vi "QEPROcontrol_version3.vi"() -> ()   [LabVIEW 2014]
uses:
  C:/Program Files (x86)/Ocean Optics/OmniDriver/OOI_HOME/NETOmniDriver-NET40.dll
  <vilib>/ptbypt/NI_PtbyPt.lvlib
panel:
  out "CV值計算\n(100個取樣點)":dbl
  out "deltaR/R":dbl(graph)
  out "deltaR/R(%)":dbl
  out "max":dbl
  out "average":dbl
  out "x-y":dbl(graph)
  out "CVP波形(1/total R)\n全光譜加總取倒數":dbl(graph)
  in  "Record Number":i32 min=0 step=1
  in  "Record?":bool
  in  "Folder Path":path
  in  "Filename":string(combo)="RAtery"
  in  "stop":bool
  out "Spectrum":cluster{"Y":dbl[], "Y":dbl[]}[](graph)
  in  "Start/Pause":bool
  in  "TEC Enable":i16(ring)=1 items=["Disable", "Enable"]
  out "Detector\nTemperature":dbl
  in  "Enter the Detector\nTemperature (C)":dbl=-18.0
  in  "Scans to Average":i32=1 min=1 max=1000000 step=1
  out "Strobe Enable":i32(ring) items=["Disable", "Enable"]
  out "NumberOfPixels":i32
  out "NumberOfDarkPixels":i32
  in  "Correct for Electrical Dark":i16(ring) items=["Disable", "Enable"]
  in  "Correct for Detector Nonlinearity":i16(ring) items=["Disable", "Enable"]
  in  "BoxcarWidth":i32 min=0 max=1052 step=1
  out "Spectrometer ID":string
  in  "Integration\nTime (s.)":dbl=0.008 caption="Integration Time (s.)" min=0.008 max=60000.0 step=0.001 format="%#.6g"
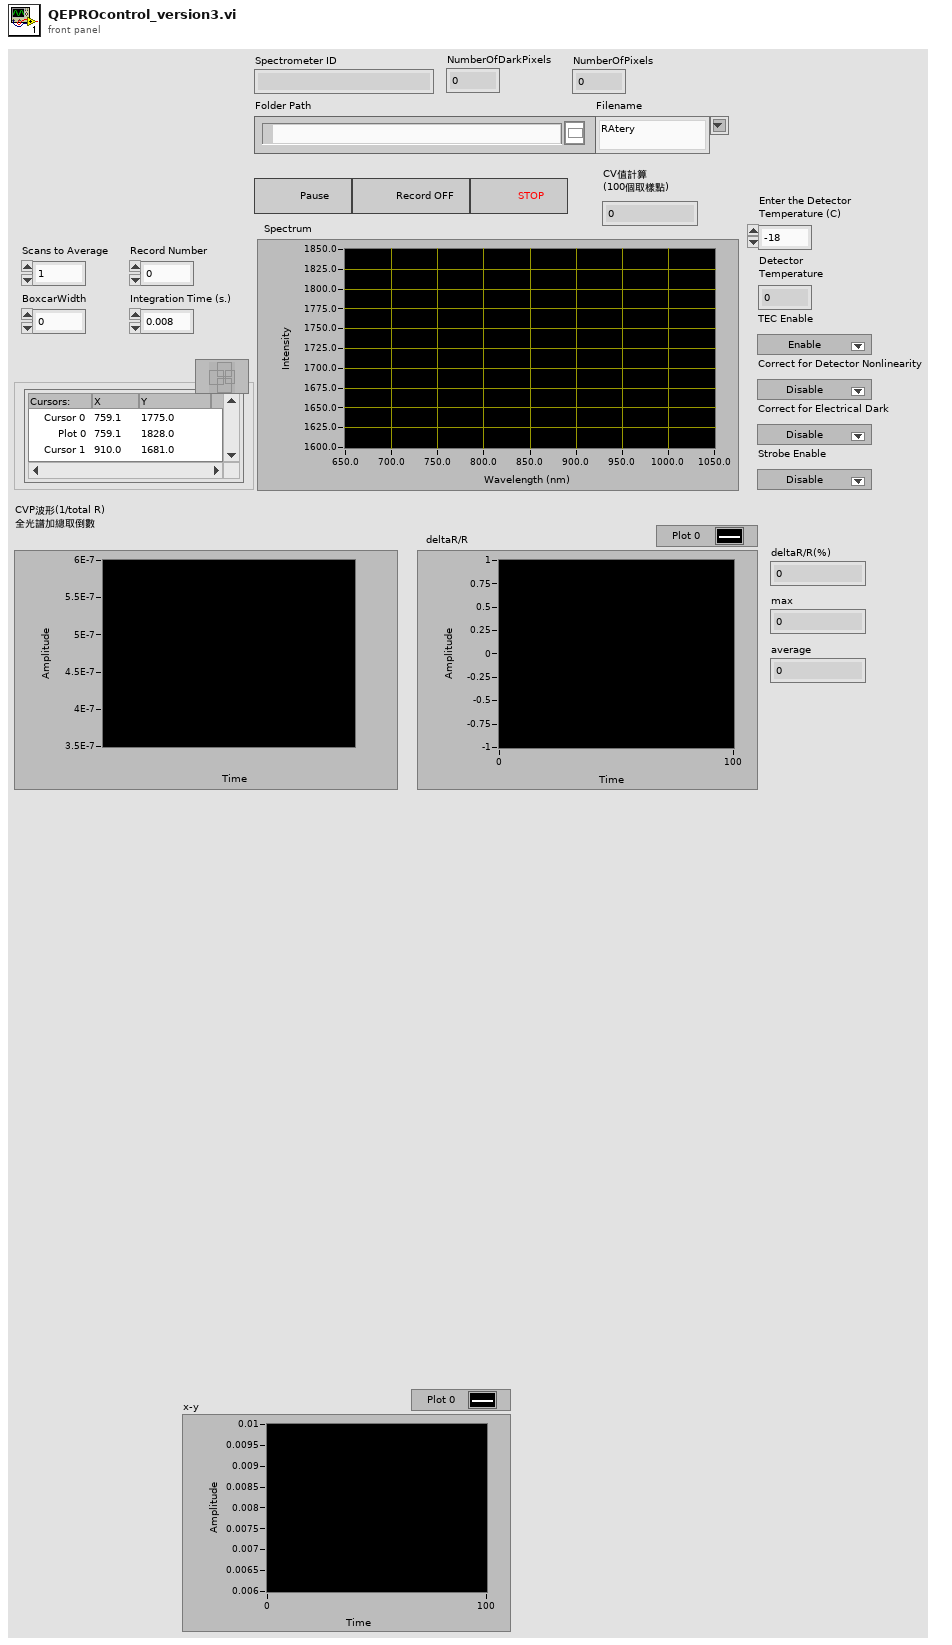
[diagram p1: front panel]
types:
  T1 = cluster{"seconds since 1Jan1904":timestamp, "getSpectrum":dbl[]}
  T2 = cluster{"seconds since 1Jan1904":timestamp, dbl[]}
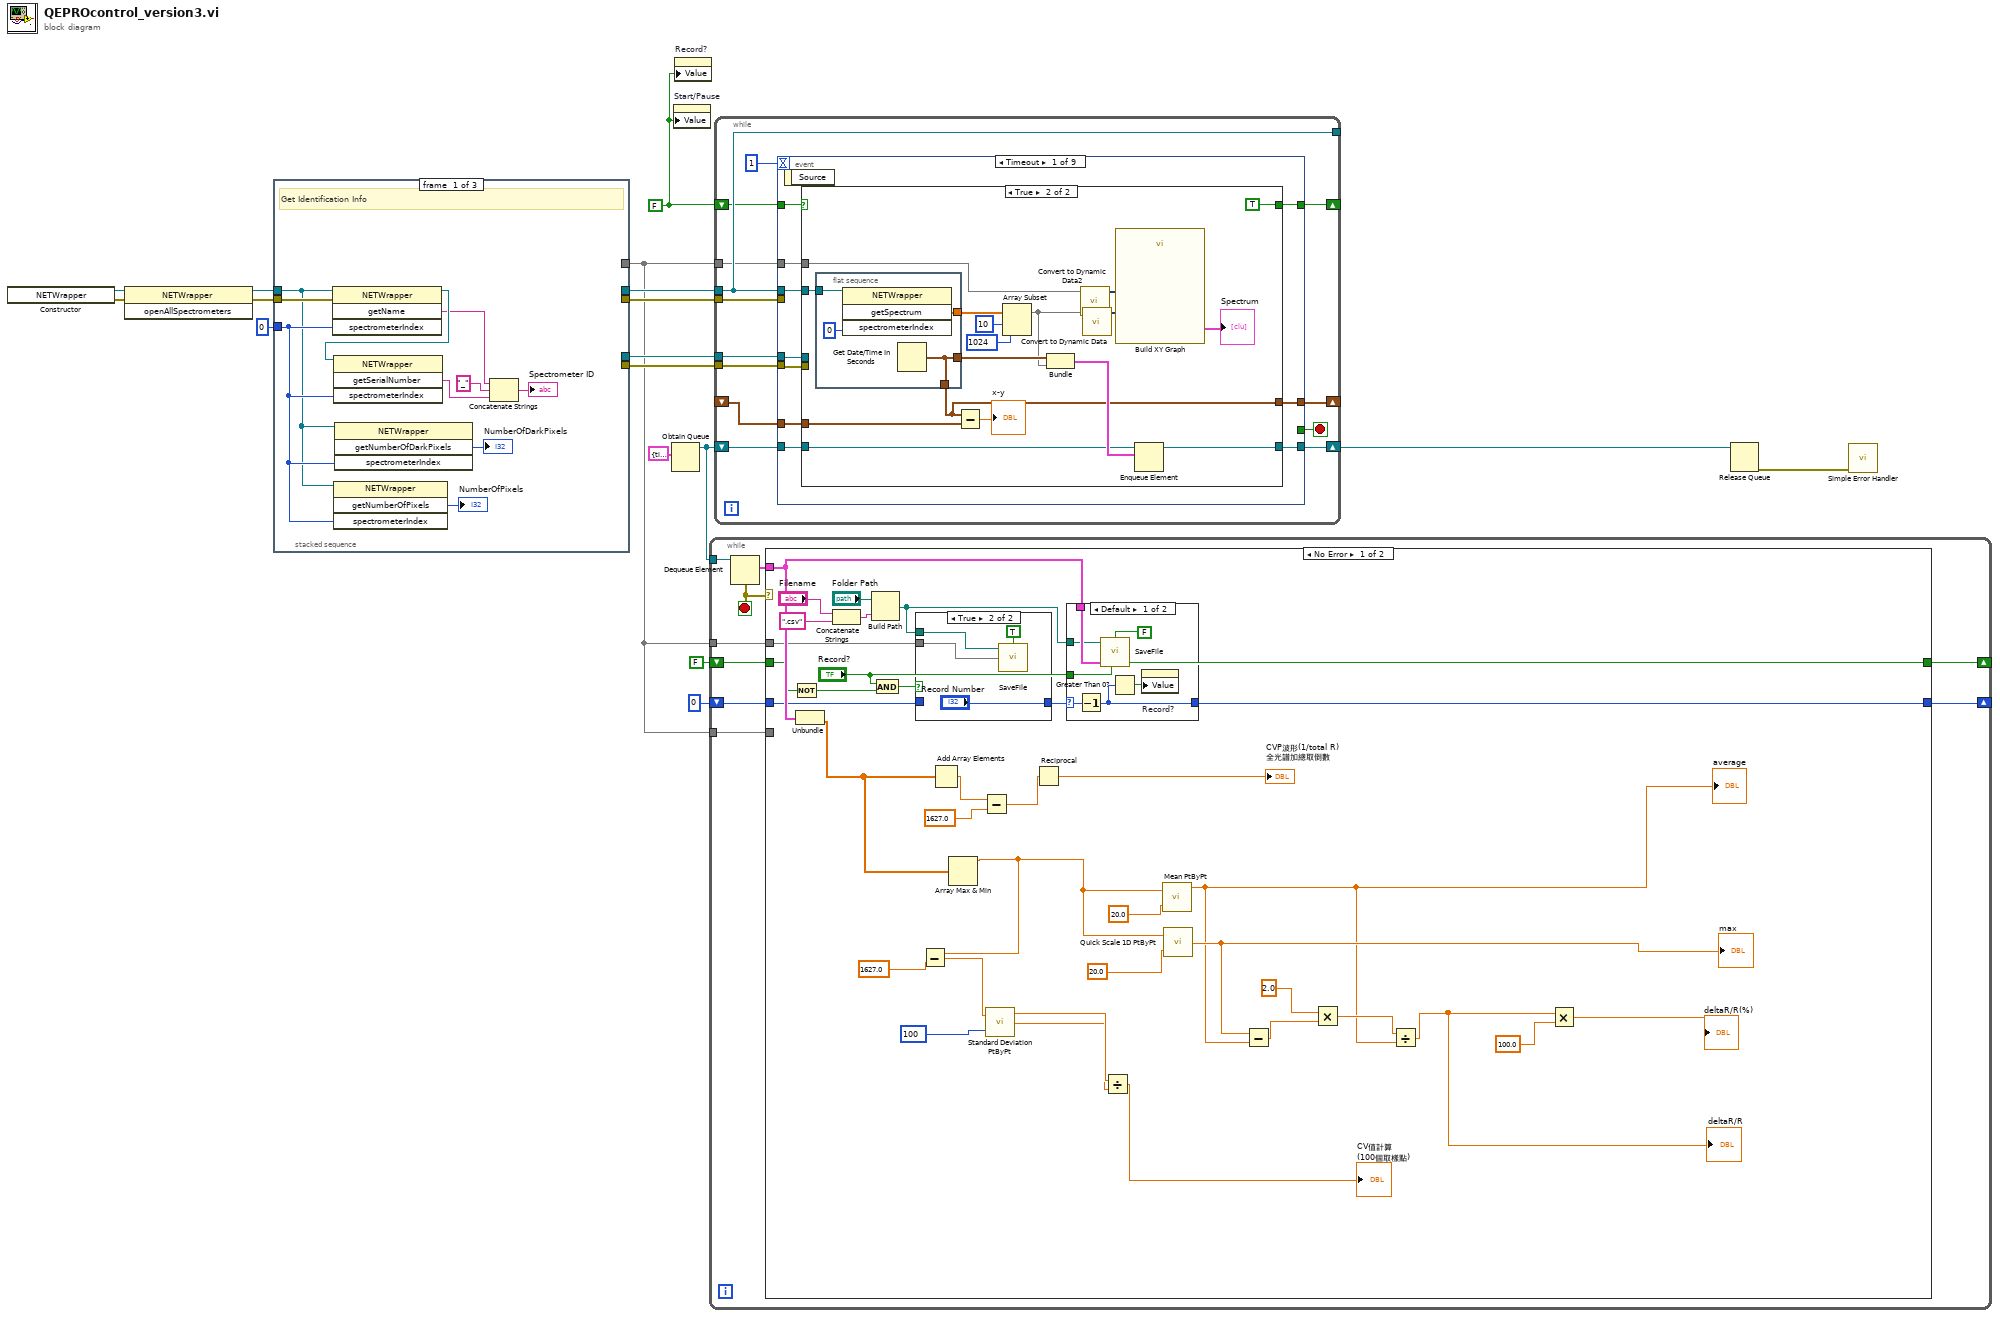
[diagram p0: block diagram]
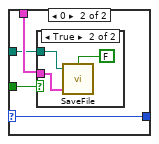
[diagram p2: hidden frame]
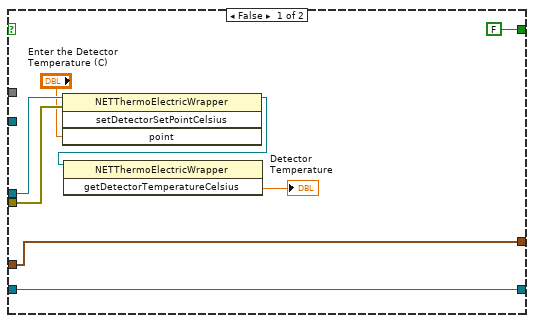
[diagram p6: hidden frame]
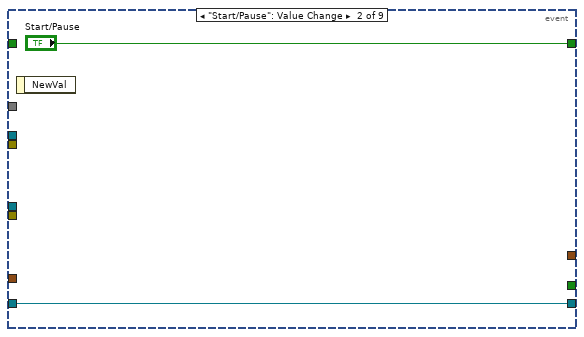
[diagram p7: hidden frame]
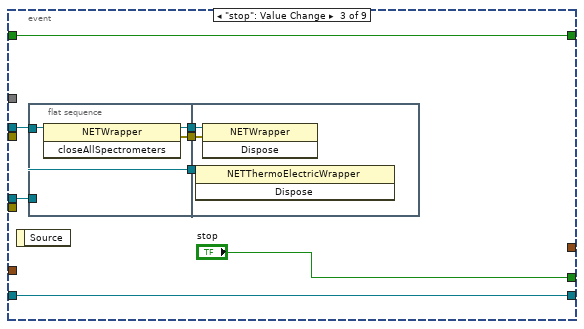
[diagram p8: hidden frame]
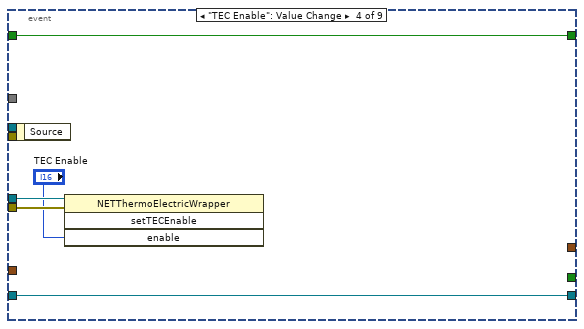
[diagram p9: hidden frame]
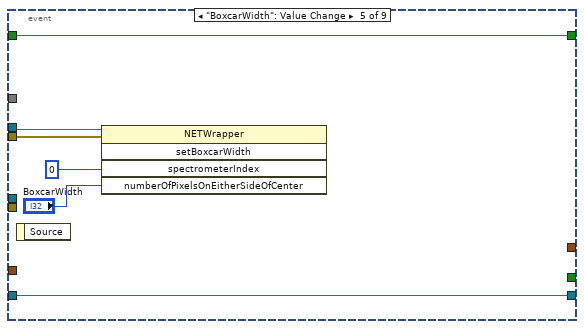
[diagram p10: hidden frame]
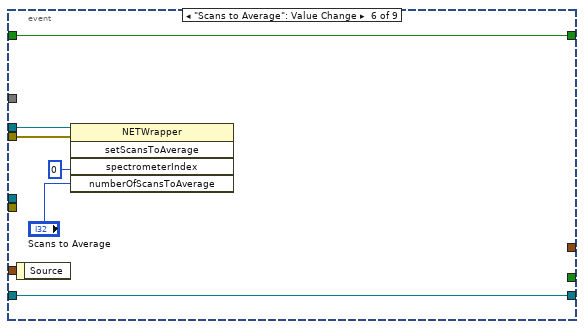
[diagram p11: hidden frame]
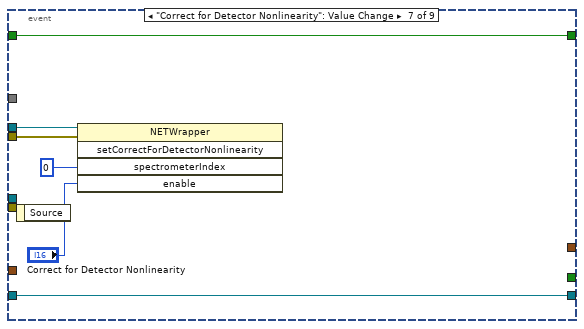
[diagram p12: hidden frame]
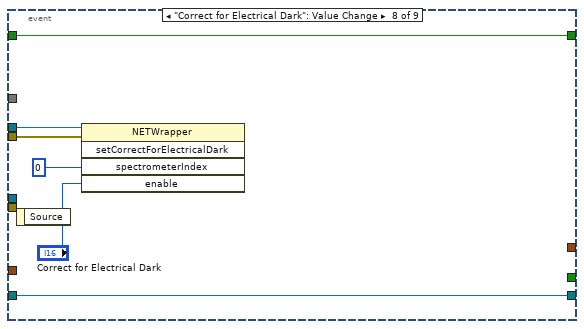
[diagram p13: hidden frame]
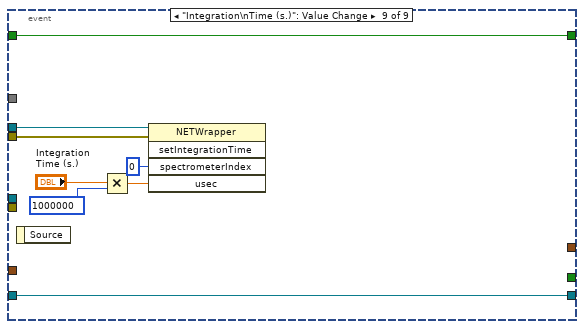
[diagram p14: hidden frame]
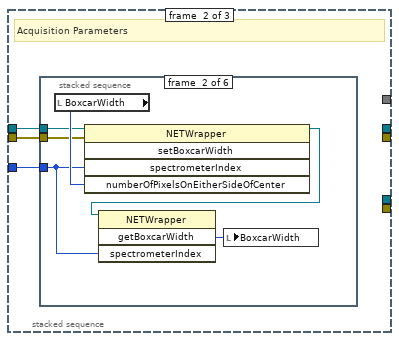
[diagram p15: hidden frame]
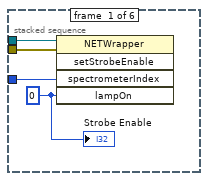
[diagram p16: hidden frame]
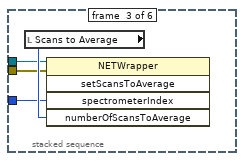
[diagram p17: hidden frame]
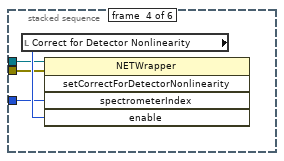
[diagram p18: hidden frame]
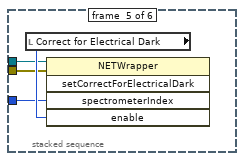
[diagram p19: hidden frame]
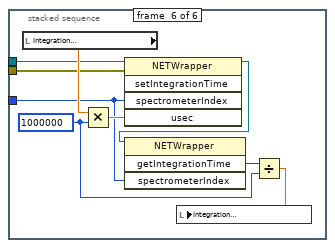
[diagram p20: hidden frame]
diagram:
  w4 = FALSE ("Start/Pause")
  n1 = constructor class="NETWrapper"() -> (reference out=w17:refnum<k24>, error out=w16:errorcluster)  [unwired: 3 in, 1 out]
  n2 = invoke class="NETWrapper" method="openAllSpectrometers"(reference=w17, error in=w16) -> (reference out=w14:refnum<k24>, error out=w13:errorcluster)  [unwired: 1 in, 1 out]
  n3 = stacked-sequence {
    tunnel: 0 ("x") -> [w21 w28 w76]
    tunnel: w14 -> [w18 w30 w77]
    tunnel: w13 -> [w22 w29 w80]
    tunnel: [_ _ w79] -> w12
    tunnel: [_ _ w72] -> w11
    tunnel: [_ _ w78] -> w10
    tunnel: [_ _ w64] -> w8
    tunnel: [_ _ w74] -> w9
    frame #0 {
      # "Get Identification Info"
      n4 = invoke class="NETWrapper" method="getName"(reference=w18, error in=w22, "spectrometerIndex"=w21) -> (reference out=w27:refnum<k24>, "getName"=w25:string)  [unwired: 1 in, 2 out]
      n5 = invoke class="NETWrapper" method="getSerialNumber"(reference=w27, "spectrometerIndex"=w21) -> ("getSerialNumber"=w24:string)  [unwired: 2 in, 3 out]
      n6 = invoke class="NETWrapper" method="getNumberOfPixels"(reference=w18, "spectrometerIndex"=w21) -> ("getNumberOfPixels"=→"NumberOfPixels":i32)  [unwired: 2 in, 3 out]
      n7 = invoke class="NETWrapper" method="getNumberOfDarkPixels"(reference=w18, "spectrometerIndex"=w21) -> ("getNumberOfDarkPixels"=→"NumberOfDarkPixels":i32)  [unwired: 2 in, 3 out]
      n8 = Concatenate Strings(w25, "_", w24) -> (→"Spectrometer ID":string)
    }
    frame #1 {
      # "Acquisition Parameters"
      n9 = stacked-sequence {
        tunnel: w28 -> [w34 w37 w43 w47 w51 w55]
        tunnel: w30 -> [w33 w36 w42 w46 w50 w54]
        tunnel: w29 -> [w32 w35 w41 w45 w49 w53]
        frame #0 {
          w31 = 0 ("lampOn")
          n10 = invoke class="NETWrapper" method="setStrobeEnable"(reference=w33, error in=w32, "spectrometerIndex"=w34, "lampOn"=w31) -> ()  [unwired: 1 in, 5 out]
          "Strobe Enable" <- w31
        }
        frame #1 {
          n11 = local read "BoxcarWidth"() -> (w40:i32)
          n12 = invoke class="NETWrapper" method="setBoxcarWidth"(reference=w36, error in=w35, "spectrometerIndex"=w37, "numberOfPixelsOnEitherSideOfCenter"=w40) -> (reference out=w39:refnum<k24>)  [unwired: 1 in, 4 out]
          n13 = invoke class="NETWrapper" method="getBoxcarWidth"(reference=w39, "spectrometerIndex"=w37) -> ("getBoxcarWidth"=w38:i32)  [unwired: 2 in, 3 out]
          n14 = local write "BoxcarWidth"(w38) -> ()
        }
        frame #2 {
          n15 = local read "Scans to Average"() -> (w44:i32)
          n16 = invoke class="NETWrapper" method="setScansToAverage"(reference=w42, error in=w41, "spectrometerIndex"=w43, "numberOfScansToAverage"=w44) -> ()  [unwired: 1 in, 5 out]
        }
        frame #3 {
          n17 = local read "Correct for Detector Nonlinearity"() -> (w48:i16)
          n18 = invoke class="NETWrapper" method="setCorrectForDetectorNonlinearity"(reference=w46, error in=w45, "spectrometerIndex"=w47, "enable"=w48) -> ()  [unwired: 1 in, 5 out]
        }
        frame #4 {
          n19 = local read "Correct for Electrical Dark"() -> (w52:i16)
          n20 = invoke class="NETWrapper" method="setCorrectForElectricalDark"(reference=w50, error in=w49, "spectrometerIndex"=w51, "enable"=w52) -> ()  [unwired: 1 in, 5 out]
        }
        frame #5 {
          w57 = 1000000
          n21 = local read "Integration\nTime (s.)"() -> (w60:dbl)
          n22 = Multiply(x=w60, y=w57) -> (x*y=w61:dbl)
          n23 = invoke class="NETWrapper" method="setIntegrationTime"(reference=w54, error in=w53, "spectrometerIndex"=w55, "usec"=w61) -> (reference out=w59:refnum<k24>)  [unwired: 1 in, 4 out]
          n24 = invoke class="NETWrapper" method="getIntegrationTime"(reference=w59, "spectrometerIndex"=w55) -> ("getIntegrationTime"=w58:i32)  [unwired: 2 in, 3 out]
          n25 = Divide(x=w58, y=w57) -> (x/y=w56:dbl)
          n26 = local write "Integration\nTime (s.)"(w56) -> ()
        }
      }
    }
    frame #2 {
      w73 = i16 1 ("enable")
      n27 = Get Date/Time In Seconds() -> (seconds since 1Jan1904=w71:timestamp)
      n28 = invoke class="NETWrapper" method="getFeatureControllerThermoElectric"(reference=w77, error in=w80, "spectrometerIndex"=w76) -> (reference out=w79:refnum<k24>, error out=w74:errorcluster, "getFeatureControllerThermoElectric"=w81:refnum<k24>)  [unwired: 1 in, 1 out]
      n29 = invoke class="NETWrapper" method="getWavelengths"(reference=w77, "spectrometerIndex"=w76) -> ("getWavelengths"=w75:dbl[])  [unwired: 2 in, 3 out]
      n30 = invoke class="NETThermoElectricWrapper" method="setTECEnable"(reference=w81, "enable"=w73) -> (reference out=w72:refnum<k24>, error out=w78:errorcluster)  [unwired: 2 in, 2 out]
      n31 = call <vilib>:"Application Directory.vi"() -> ("Application Directory"=w66:path)
      n32 = Format Date/Time String(time format string (%c)="%Y%m%d", seconds (now)=w71) -> (date/time string=w69:string)  [unwired: 1 in]
      n33 = local write "TEC Enable"(w73) -> ()
      n34 = Build Path(base path=w66, name or relative path=w69) -> (appended path=w65:path)
      n35 = call <vilib>:"Check if File or Folder Exists.vi"("path"=w65) -> ("file or folder exists?"=w67:bool, "dup path"=w68:path)  [unwired: 8 in, 1 out]
      n36 = Array Subset(array=w75, index=10, length=1024 ("index")) -> (w64:dbl[])
      n37 = case shown="True" w67 {
        tunnel: w68 -> [w82 _]
        frame False {
          n38 = Create Folder(path (use dialog)=w82) -> ()  [unwired: 2 in, 3 out]
        }
        frame True {
        }
      }
      n39 = property on="Folder Path" class="Path"("Value"=w65) -> ()  [unwired: 2 in, 2 out]
    }
  }
  n40 = Obtain Queue(element data type=T1 {"seconds since 1Jan1904"=timestamp(0 s since 1904-01-01), "getSpectrum"=[]} ("output cluster")) -> (queue out=w5:refnum<queue>)  [unwired: 4 in, 2 out]
  n41 = property on="Start/Pause" class="Bool (strict)"("Value"=w4) -> ()  [unwired: 2 in, 2 out]
  n42 = property on="Record?" class="Bool (strict)"("Value"=w4) -> ()  [unwired: 2 in, 2 out]
  n43 = while {
    tunnel: w5 -> [w91]
    shift-right: [w88] -> _
    shift-left: FALSE ("Rec?") -> [w89]
    tunnel: w8 -> [w87]
    shift-right: [w84] -> _
    shift-left: 0 -> [w85]
    tunnel: w8 -> [w83]
    stop <- w86 stop-if-true
    n44 = Dequeue Element(queue=w91) -> (element=w90:T1, error out=w86:errorcluster)  [unwired: 2 in, 2 out]
    n45 = case shown="No Error" w86 {
      tunnel: w90 -> [w127 _]
      tunnel: w89 -> [w122 w146]
      tunnel: ["Record?" w146] -> w88
      tunnel: w87 -> [w119 _]
      tunnel: w85 -> [w118 w147]
      tunnel: [w116 w147] -> w84
      tunnel: w83 -> [_ _]
      frame No Error {
        n46 = Not(x=w122) -> (.not. x?=w121:bool)
        n47 = Unbundle(w127) -> ("getSpectrum"=w93:dbl[])  [unwired: 1 out]
        n48 = Concatenate Strings("Filename", ".csv" ("string")) -> (w126:string)
        n49 = Build Path(base path="Folder Path", name or relative path=w126) -> (appended path=w117:path)
        n50 = And(x="Record?", y=w121) -> (x .and. y?=w120:bool)
        n51 = case shown="True" w120 {
          tunnel: w119 -> [_ w144]
          tunnel: w117 -> [_ w143]
          tunnel: [w141 "Record Number"] -> w114
          tunnel: w118 -> [w141 _]
          frame False {
          }
          frame True {
            n52 = call "SaveFile.vi"("First call?"=TRUE, "Wavelengths"=w144, "Path"=w143) -> ()  [unwired: 2 in]
          }
        }
        n53 = Add Array Elements(numeric array=w93) -> (sum=w102:dbl)
        n54 = Array Max & Min(array=w93) -> (max value=w94:dbl)  [unwired: 3 out]
        n55 = Subtract(x=w94, y=1627.0) -> (x-y=w98:dbl)
        n56 = Subtract(x=w102, y=1627.0) -> (x-y=w92:dbl)
        n57 = call <vilib>:"Standard Deviation PtByPt.vi"("x"=w98, "sample length"=100) -> ("standard deviation"=w97:dbl, "mean"=w96:dbl)  [unwired: 1 in, 1 out]
        n58 = Reciprocal(x=w92) -> (1/x=→"CVP波形(1/total R)\n全光譜加總取倒數":dbl)
        n59 = case shown="Default" w114 {
          selector: w114 -> [w133 w134]
          tunnel: w127 -> [w131 w136]
          tunnel: w117 -> [w130 w135]
          tunnel: [w128 w134] -> w116
          tunnel: "Record?" -> [_ w137]
          frame Default {
            n60 = Decrement(x=w133) -> (x-1=w128:i32)
            n61 = call "SaveFile.vi"("First call?"=FALSE, "time Spectrum"=w131, "Path"=w130) -> ()  [unwired: 2 in]
            n62 = Greater Than 0?(x=w128) -> (x > 0?=w132:bool)
            n63 = property on="Record?" class="Bool (strict)"("Value"=w132) -> ()  [unwired: 2 in, 2 out]
          }
          frame 0 {
            n64 = case shown="True" w137 {
              tunnel: w136 -> [_ w138]
              tunnel: w135 -> [_ w140]
              frame False {
              }
              frame True {
                n65 = call "SaveFile.vi"("First call?"=FALSE, "time Spectrum"=w138, "Path"=w140) -> ()  [unwired: 2 in]
              }
            }
          }
        }
        n66 = Divide(x=w97, y=w96) -> (x/y=→"CV值計算\n(100個取樣點)":dbl)
        n67 = call <vilib>:"Mean PtByPt.vi"("x"=w94, "sample length"=20.0 ("x*y")) -> ("mean"=w108:dbl)  [unwired: 2 in, 1 out]
        "average" <- w108
        n68 = call <vilib>:"Quick Scale 1D PtByPt.vi"("x"=w94, "sample length"=20.0 ("x*y")) -> ("max|X|"=w112:dbl)  [unwired: 1 in, 2 out]
        "max" <- w112
        n69 = Subtract(x=w112, y=w108) -> (x-y=w111:dbl)
        n70 = Multiply(x=2.0 ("x*y"), y=w111) -> (x*y=w109:dbl)
        n71 = Divide(x=w109, y=w108) -> (x/y=w104:dbl)
        "deltaR/R" <- w104
        n72 = Multiply(x=w104, y=100.0) -> (x*y=→"deltaR/R(%)":dbl)
      }
      frame Error {
      }
    }
  }
  n73 = while {
    tunnel: w12 -> [w159]
    tunnel: w11 -> [w158]
    tunnel: w10 -> [w160]
    tunnel: [w159] -> _
    tunnel: w9 -> [w157]
    shift-right: [w154] -> _
    shift-left: w4 -> [w153]
    tunnel: w8 -> [w152]
    shift-right: [w150] -> w6
    shift-left: w5 -> [w151]
    shift-right: [w149] -> _
    shift-left: _ -> [w148]
    stop <- w155 stop-if-true
    n74 = event shown="[0] Timeout" {
      selector: _ -> [_ _ _ _ _ _ _ _ _]
      dyn-events: _ -> [_ _ _ _ _ _ _ _ _]
      timeout: 1 -> [_ _ _ _ _ _ _ _ _]
      tunnel: w159 -> [w167 _ w206 _ w227 w233 w239 w245 w250]
      tunnel: w158 -> [w170 _ w205 w221 _ _ _ _ _]
      tunnel: w160 -> [w169 _ _ w220 _ _ _ _ _]
      tunnel: w157 -> [_ _ _ _ w224 w232 w236 w242 w248]
      tunnel: [_ _ "stop" _ _ _ _ _ _] -> w155
      tunnel: [w163 "Start/Pause" w202 w217 w222 w228 w234 w240 w246] -> w154
      tunnel: w153 -> [w168 _ w202 w217 w222 w228 w234 w240 w246]
      tunnel: w152 -> [w166 _ _ _ _ _ _ _ _]
      tunnel: w151 -> [w165 w200 w203 w218 w223 w229 w235 w241 w247]
      tunnel: [w164 w200 w203 w218 w223 w229 w235 w241 w247] -> w150
      tunnel: [w162 _ _ _ _ _ _ _ _] -> w149
      tunnel: w148 -> [w161 _ _ _ _ _ _ _ _]
      event Timeout {
        n75 = event-data() -> ()  [unwired: 1 in, 1 out]
        n76 = case shown="True" w168 {
          tunnel: w170 -> [w178 _]
          tunnel: w169 -> [w177 _]
          tunnel: w167 -> [_ w192]
          tunnel: w166 -> [_ w191]
          tunnel: w165 -> [w173 w187]
          tunnel: [w173 w186] -> w164
          tunnel: [FALSE ("Start/Pause") TRUE ("Start/Pause")] -> w163
          tunnel: [w171 w181] -> w162
          tunnel: w161 -> [w171 w180]
          frame False {
            n77 = invoke class="NETThermoElectricWrapper" method="setDetectorSetPointCelsius"(reference=w178, error in=w177, "point"="Enter the Detector\nTemperature (C)") -> (reference out=w174:refnum<k24>)  [unwired: 1 in, 3 out]
            n78 = invoke class="NETThermoElectricWrapper" method="getDetectorTemperatureCelsius"(reference=w174) -> ("getDetectorTemperatureCelsius"=→"Detector\nTemperature":dbl)  [unwired: 2 in, 2 out]
          }
          frame True {
            n79 = flat-sequence {
              tunnel: [w198] -> w190
              tunnel: [w196] -> w189
              tunnel: w192 -> [w197]
              tunnel: [w196] -> w181
              frame #0 {
                n80 = invoke class="NETWrapper" method="getSpectrum"(reference=w197, "spectrometerIndex"=0) -> ("getSpectrum"=w198:dbl[])  [unwired: 2 in, 3 out]
                n81 = Get Date/Time In Seconds() -> (seconds since 1Jan1904=w196:timestamp)
              }
            }
            n82 = Subtract(x=w181, y=w180) -> (x-y=→"x-y":dbl)
            n83 = Array Subset(array=w190, index=10, length=1024 ("index")) -> (w183:dbl[])
            n84 = Bundle("seconds since 1Jan1904"=w189, w183) -> (w188:T2)  [unwired: 1 in]
            n85 = call "Convert to Dynamic Data2"("Array"=w191) -> ("Dynamic Data Type"=w193:dynamicdata)  [unwired: 3 in]
            n86 = call "Convert to Dynamic Data"("Array"=w183) -> ("Dynamic Data Type"=w195:dynamicdata)  [unwired: 3 in]
            n87 = call "Build XY Graph"("Y Input"=w195, "X Input"=w193) -> ("XY Graph"=→"Spectrum":cluster{"Y":dbl[], "Y":dbl[]}[])  [unwired: 8 in, 1 out]
            n88 = Enqueue Element(queue=w187, element=w188) -> (queue out=w186:refnum<queue>)  [unwired: 2 in, 2 out]
          }
        }
      }
      event "Start/Pause": Value Change {
        n89 = event-data() -> ()  [unwired: 1 in, 1 out]
      }
      event "stop": Value Change {
        n90 = event-data() -> ()  [unwired: 1 in, 1 out]
        n91 = flat-sequence {
          tunnel: [w213] -> w209
          tunnel: [w212] -> w208
          tunnel: [w210] -> w207
          tunnel: w206 -> [w211]
          tunnel: w205 -> [w210]
          tunnel: w209 -> [w216]
          tunnel: w208 -> [w215]
          tunnel: w207 -> [w214]
          frame #0 {
            n92 = invoke class="NETWrapper" method="closeAllSpectrometers"(reference=w211) -> (reference out=w213:refnum<k24>, error out=w212:errorcluster)  [unwired: 2 in, 1 out]
          }
          frame #1 {
            n93 = invoke class="NETThermoElectricWrapper" method="Dispose"(reference=w214) -> ()  [unwired: 2 in, 3 out]
            n94 = invoke class="NETWrapper" method="Dispose"(reference=w216, error in=w215) -> ()  [unwired: 1 in, 3 out]
          }
        }
      }
      event "TEC Enable": Value Change {
        n95 = event-data() -> ()  [unwired: 1 in, 1 out]
        n96 = invoke class="NETThermoElectricWrapper" method="setTECEnable"(reference=w221, error in=w220, "enable"="TEC Enable") -> ()  [unwired: 1 in, 4 out]
      }
      event "BoxcarWidth": Value Change {
        n97 = event-data() -> ()  [unwired: 1 in, 1 out]
        n98 = invoke class="NETWrapper" method="setBoxcarWidth"(reference=w227, error in=w224, "spectrometerIndex"=0, "numberOfPixelsOnEitherSideOfCenter"="BoxcarWidth") -> ()  [unwired: 1 in, 5 out]
      }
      event "Scans to Average": Value Change {
        n99 = event-data() -> ()  [unwired: 1 in, 1 out]
        n100 = invoke class="NETWrapper" method="setScansToAverage"(reference=w233, error in=w232, "spectrometerIndex"=0, "numberOfScansToAverage"="Scans to Average") -> ()  [unwired: 1 in, 5 out]
      }
      event "Correct for Detector Nonlinearity": Value Change {
        n101 = event-data() -> ()  [unwired: 1 in, 1 out]
        n102 = invoke class="NETWrapper" method="setCorrectForDetectorNonlinearity"(reference=w239, error in=w236, "spectrometerIndex"=0, "enable"="Correct for Detector Nonlinearity") -> ()  [unwired: 1 in, 5 out]
      }
      event "Correct for Electrical Dark": Value Change {
        n103 = event-data() -> ()  [unwired: 1 in, 1 out]
        n104 = invoke class="NETWrapper" method="setCorrectForElectricalDark"(reference=w245, error in=w242, "spectrometerIndex"=0, "enable"="Correct for Electrical Dark") -> ()  [unwired: 1 in, 5 out]
      }
      event "Integration\nTime (s.)": Value Change {
        n105 = event-data() -> ()  [unwired: 1 in, 1 out]
        n106 = Multiply(x="Integration\nTime (s.)", y=1000000) -> (x*y=w251:dbl)
        n107 = invoke class="NETWrapper" method="setIntegrationTime"(reference=w250, error in=w248, "spectrometerIndex"=0, "usec"=w251) -> ()  [unwired: 1 in, 5 out]
      }
    }
  }
  n108 = Release Queue(queue=w6) -> (error out=w3:errorcluster)  [unwired: 2 in, 2 out]
  n109 = call <vilib>:"Simple Error Handler.vi"("error in (no error)"=w3) -> ()  [unwired: 4 in, 5 out]
